vi "Check Score Over.vi"(8 "error in (no error)":errorcluster, 11 "Game Board in":refnum<class "Game Board.lvclass">) -> (2 "Score over?":bool)   [LabVIEW 2024, in "Game Board.lvclass"]
doc: "MIT Licence\nCopyright (c) 2024 David Grollier"
uses:
  Game Board.lvclass
  Game Board.lvclass/Game Board.ctl
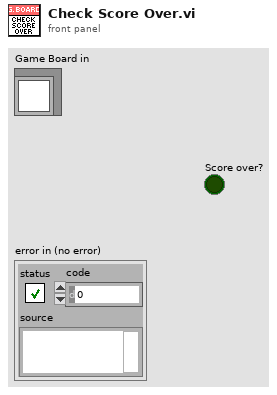
[diagram p1: front panel]
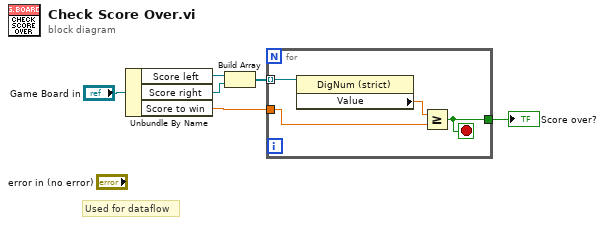
[diagram p0: block diagram]
diagram:
  # "Used for dataflow"
  n1 = Unbundle By Name("Game Board in") -> ("Score left"=w6:refnum<vi>, "Score right"=w5:refnum<vi>, "Score to win"=w3:dbl)
  n2 = Build Array(w6, w5) -> (w4:refnum<vi>[])
  n3 = for {
    tunnel: w4 -> [w10] mode=indexing
    tunnel: w3 -> [w8]
    tunnel: [w7] -> w1
    stop <- w7 stop-if-true
    n4 = property class="DigNum (strict)"(reference=w10) -> ("Value"=w9:dbl)  [unwired: 1 in, 2 out]
    n5 = Greater Or Equal?(x=w9, y=w8) -> (x >= y?=w7:bool)
  }
  "Score over?" <- w1
